vi "3654Drive2018.vi"(6 "turbo 2":bool, 7 "turbo 1":bool, 8 "Joystick2y":dbl, 9 "Joystick2x":dbl, 10 "joystick y":dbl, 11 "joystick x":dbl) -> ()   [LabVIEW 2017]
uses:
  <vilib>/Rock Robotics/WPI/ThirdParty/Phoenix-LabVIEW/Motor Controller/Controls/CTRE_Phoenix_MotorControl_ControlMode.ctl
  Robot Global Data.vi
  <vilib>/Rock Robotics/WPI/ThirdParty/Phoenix-LabVIEW/Motor Controller/Get/CTRE_Phoenix_MotorController_GetOutputCurrent_Enhanced.vi
  <vilib>/Rock Robotics/WPI/ThirdParty/Phoenix-LabVIEW/Motor Controller/Get/CTRE_Phoenix_MotorController_GetSelectedSensorData.vi
  <vilib>/Rock Robotics/WPI/ThirdParty/Phoenix-LabVIEW/Motor Controller/Get/CTRE_Phoenix_MotorController_GetClosedLoopData.vi
  <vilib>/Rock Robotics/WPI/ThirdParty/Phoenix-LabVIEW/Motor Controller/Get/CTRE_Phoenix_MotorController_GetVoltage.vi
panel:
  out "LeftCurrent":dbl
  out "RightCurrent":dbl
  out "RightClosed-loop Error":i32
  out "RightClosed-loop Target":i32
  out "LeftClosed-loop Error":i32
  out "LeftClosed-loop Target":i32
  out "RightSensorPosRotations":i32
  out "Motor output Plot 2":cluster{"Applied Throttle":dbl}(graph)
  out "RightTarget RPM":dbl
  out "RightSensorRPM Velocity RPM":i32
  out "RightApplied Output":dbl
  out "LeftSensorPosRotation":i32
  out "Motor output Plot":cluster{"Applied Throttle":dbl}(graph)
  out "LeftTarget RPM":dbl
  out "LeftSensorRPM Velocity RPM":i32
  out "LeftApplied Output":dbl
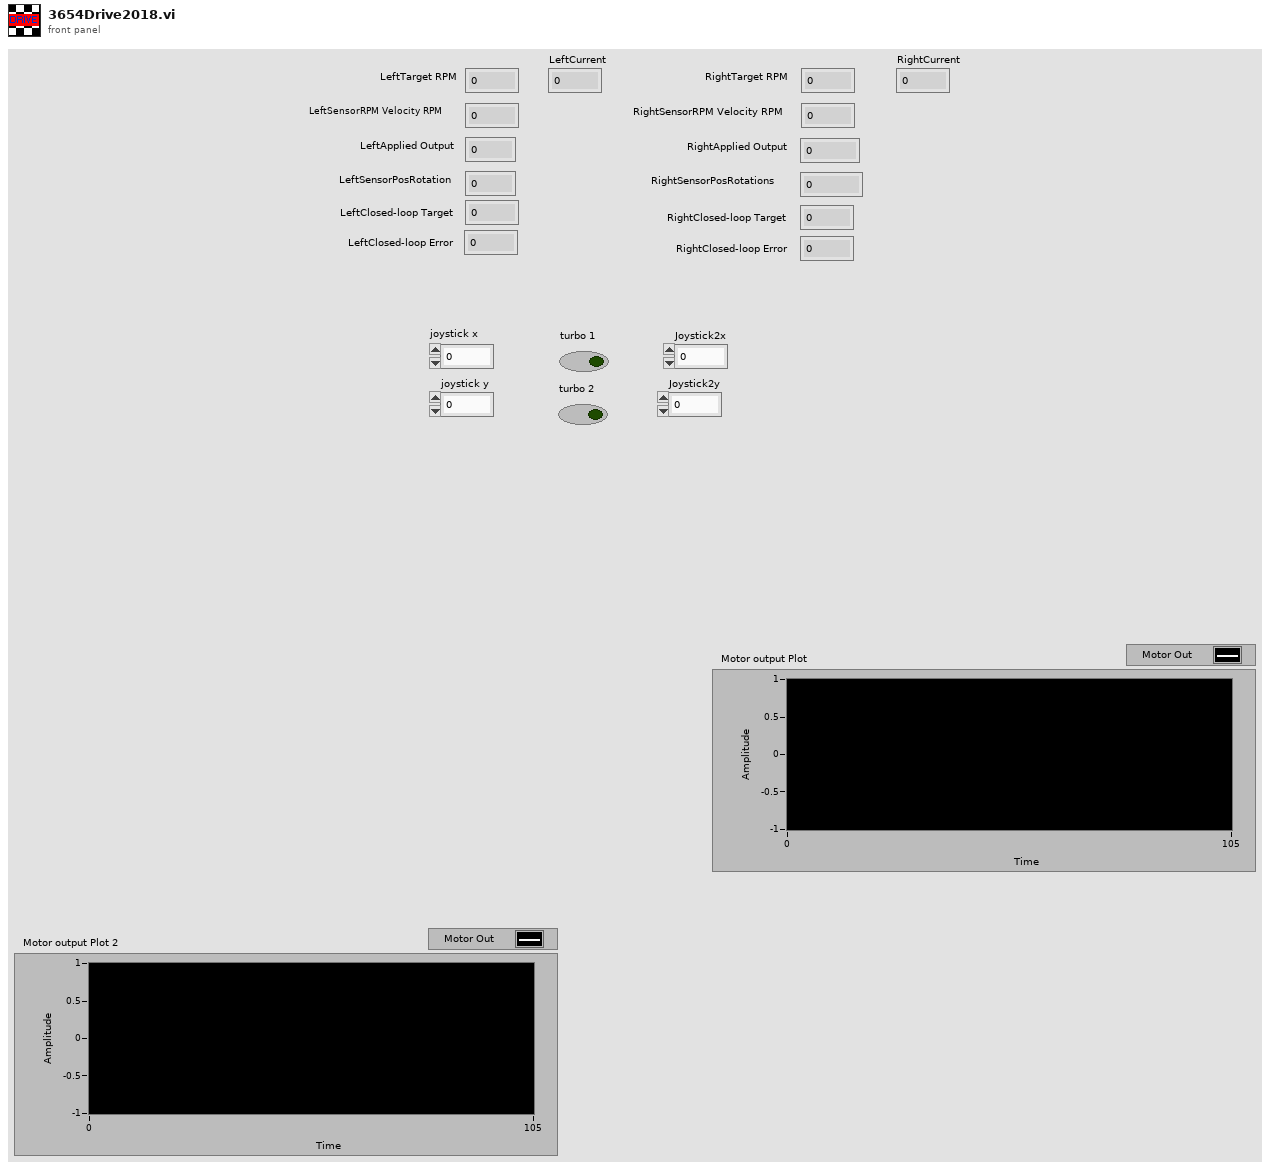
[diagram p1: front panel]
types:
  T1 = typedef "Encoder.ctl" = enum16{"NoEncoders", "ShaftEncoders", "MotorEncoders"}
  T2 = typedef "CTRE_Phoenix_MotorControl_ControlMode.ctl" = u16
  T3 = typedef "WPI_MotorControlDeviceRef.ctl" = cluster{"DeviceStatus":errorcluster, "Type":T4, "PWM":cluster{"PWM Channel":T5, "DeadBand":T6}, "CAN":cluster{"Device Number":u8, "SetOutput VI Ref":variant, "GetOutput VI Ref":variant, "Enable VI Ref":variant, "Disable VI Ref":variant, "Data":variant}, "Invert":bool, "DIO PWM":cluster{"PWM \"Enable\" Channel":T5, "DIOChannel":T7, "PWM Rate":dbl}}
  T4 = typedef "WPI_MotorControlType.ctl" = enum16{"PWM", "CAN", "DIO PWM"}
  T5 = typedef "FPGA_DIOPWMChannel.ctl" = enum8{"PWM 0", "PWM 1", "PWM 2", "PWM 3", "PWM 4", "PWM 5", "PWM 6", "PWM 7", "PWM 8", "PWM 9", "PWM MXP 0", "PWM MXP 1", "PWM MXP 2", "PWM MXP 3", "PWM MXP 4", "PWM MXP 5", "PWM MXP 6", "PWM MXP 7", "PWM MXP 8", "PWM MXP 9", "Invalid"}
  T6 = typedef "WPI_PWMDeadband.ctl" = cluster{"Name":string, "maxPositivePwm":i32, "minPositivePwm":i32, "centerPwm":i32, "maxNegativePwm":i32, "minNegativePwm":i32, "angularRange":u16}
  T7 = typedef "FPGA_DIOChannel.ctl" = enum8{"DIO 0", "DIO 1", "DIO 2", "DIO 3", "DIO 4", "DIO 5", "DIO 6", "DIO 7", "DIO 8", "DIO 9", "DIO MXP 0", "DIO MXP 1", "DIO MXP 2", "DIO MXP 3", "DIO MXP 4", "DIO MXP 5", "DIO MXP 6", "DIO MXP 7", "DIO MXP 8", "DIO MXP 9", "DIO MXP 10", "DIO MXP 11", "DIO MXP 12", "DIO MXP 13", "DIO MXP 14", "DIO MXP 15", "SPI Port CS1", "SPI Port CS2", "SPI Port CS3", "SPI Port MISO", "SPI Port MOSI", "Invalid"}
  T8 = typedef "DriveMode.ctl" = enum16{"1JoystickArcade", "2JoystickArcade", "Tank"}
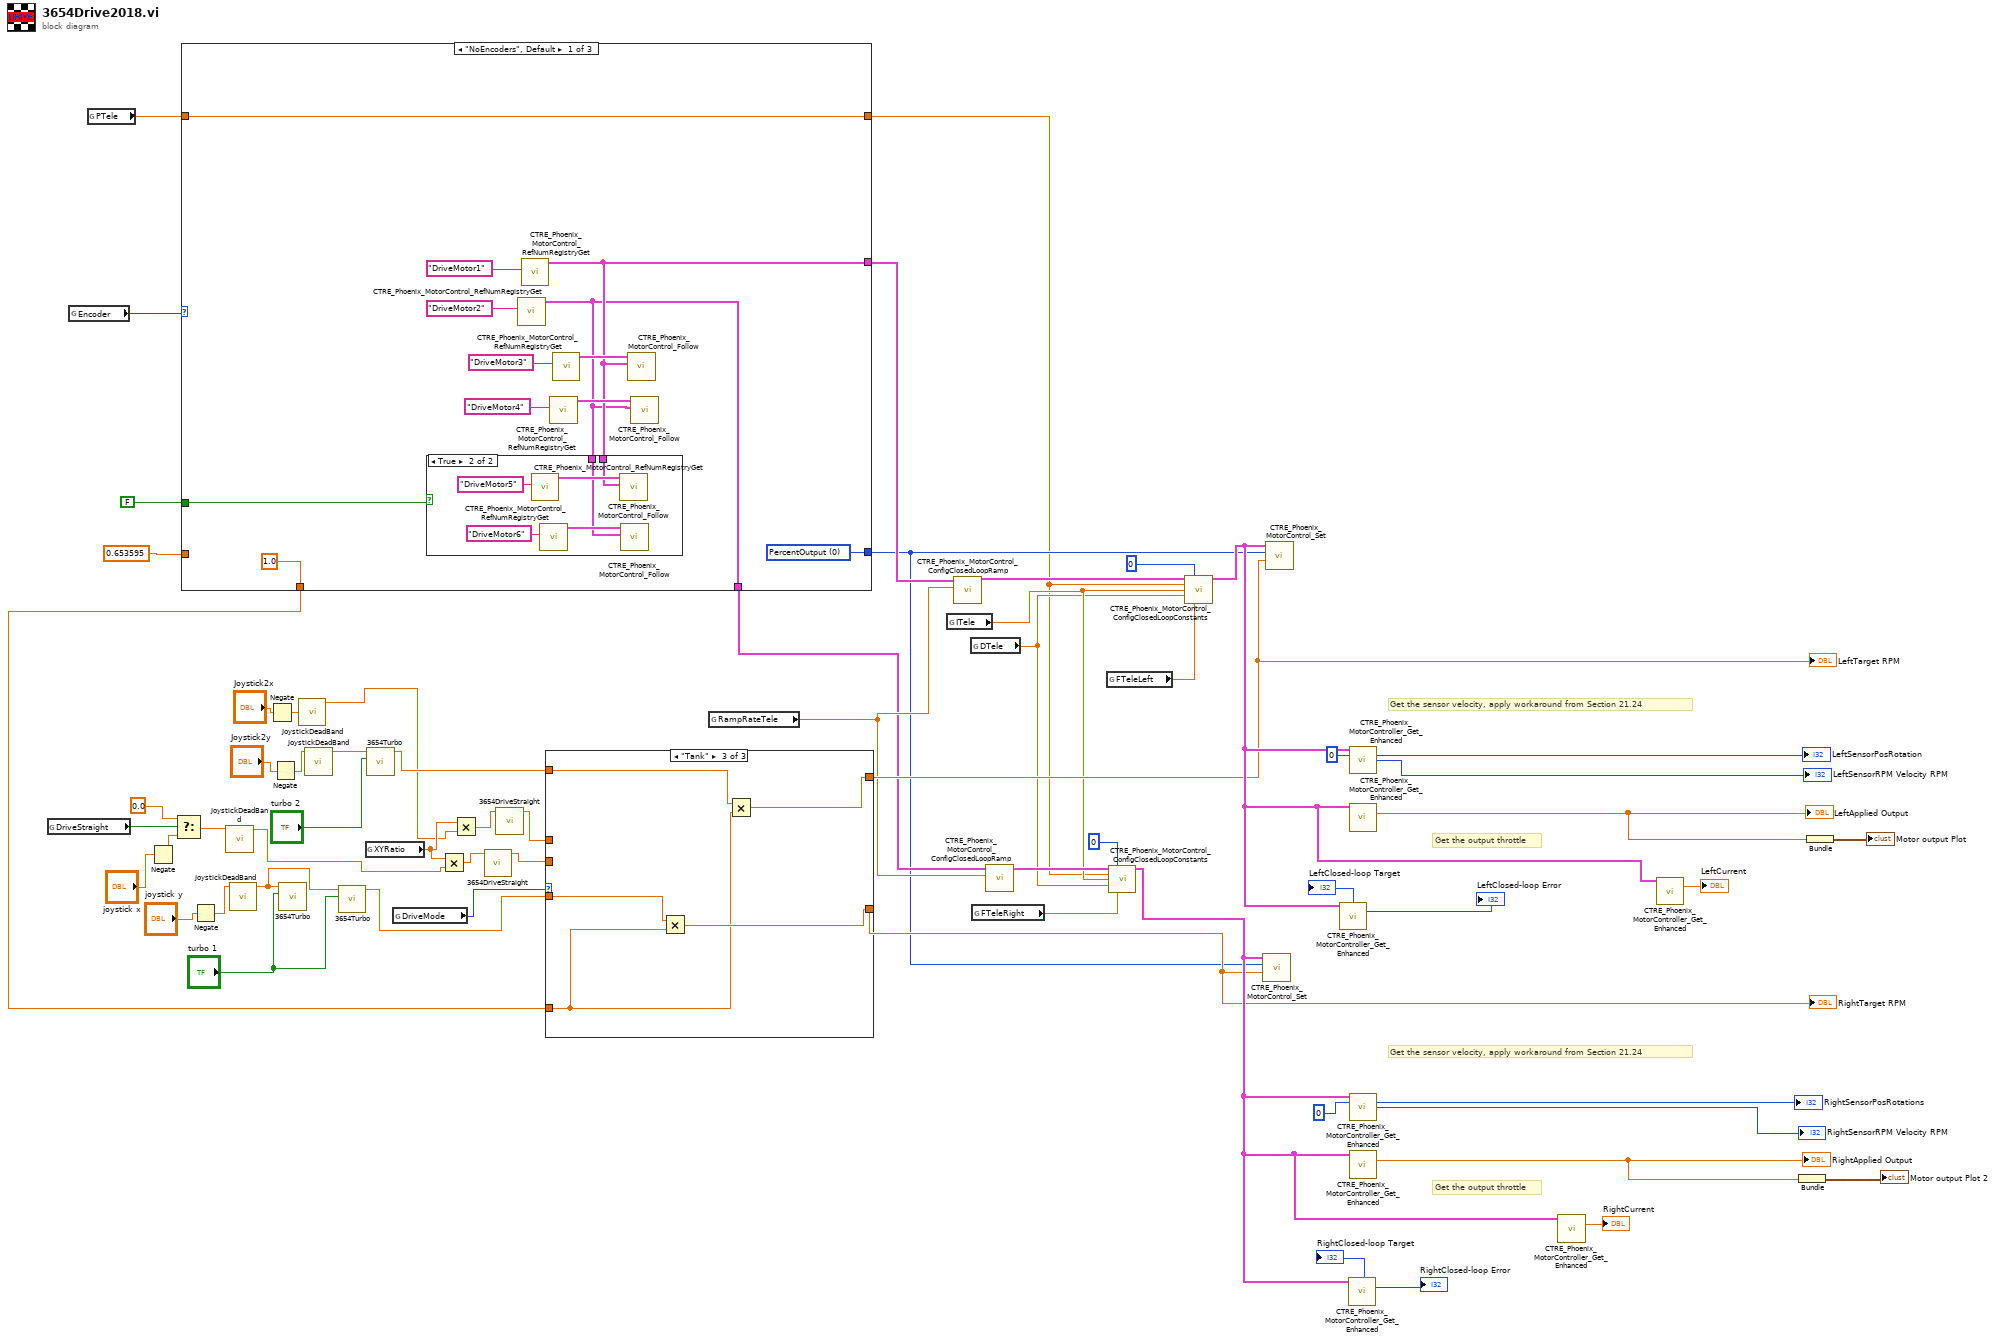
[diagram p0: block diagram]
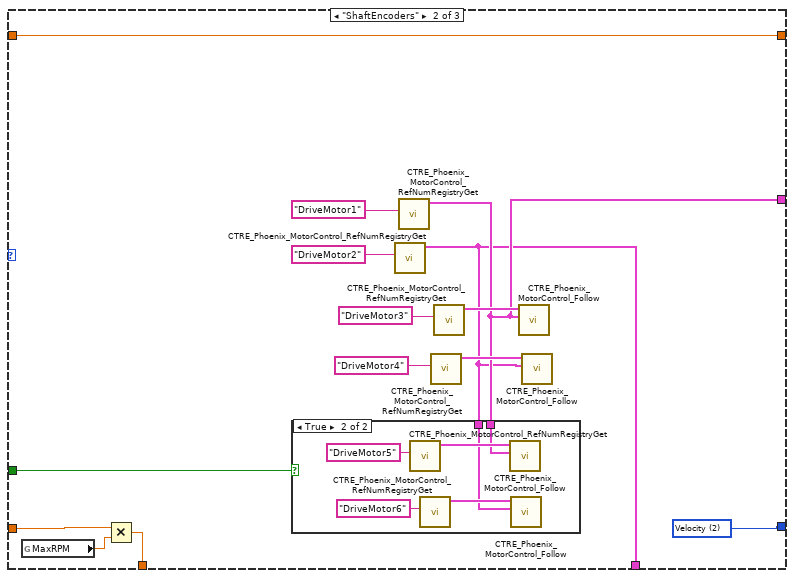
[diagram p3: hidden frame]
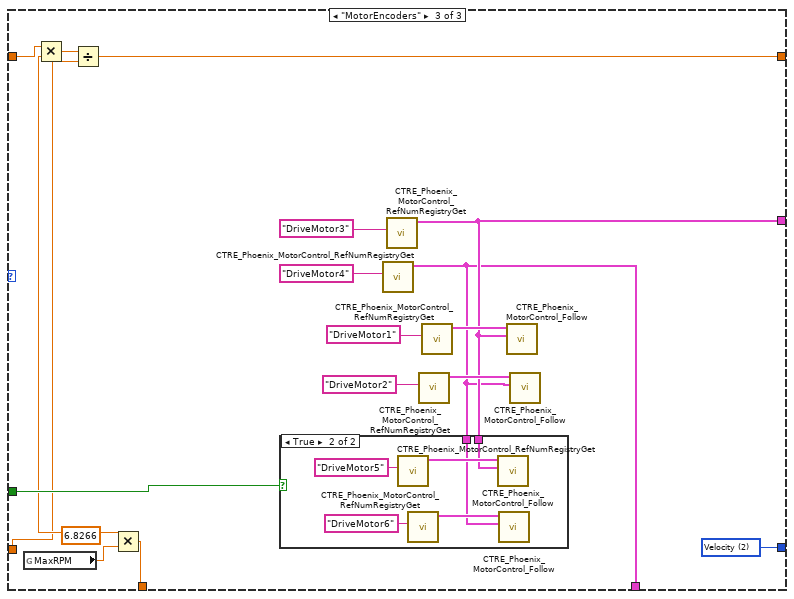
[diagram p5: hidden frame]
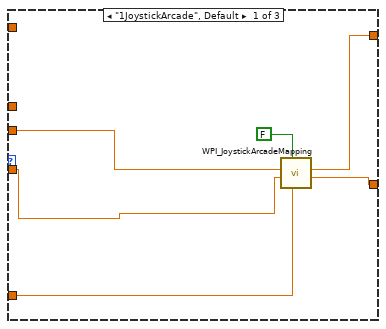
[diagram p7: hidden frame]
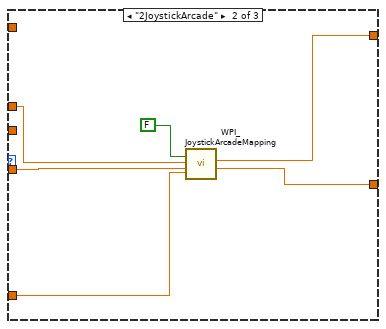
[diagram p8: hidden frame]
diagram:
  # "Get the output throttle"
  # "Get the sensor velocity, apply workaround from Section 21.24"
  # "Get the output throttle"
  # "Get the sensor velocity, apply workaround from Section 21.24"
  n1 = global read "Robot Global Data.vi" "DriveStraight"() -> (w41:bool)
  n2 = global read "Robot Global Data.vi" "Encoder"() -> (w10:T1)
  n3 = global read "Robot Global Data.vi" "PTele"() -> (w3:dbl)
  n4 = Negate(x="joystick x") -> (-x=w32:dbl)
  n5 = Select(t=0.0, s=w41, f=w32) -> (s? t:f=w40:dbl)
  n6 = case shown="\"NoEncoders\", Default" w10 {
    tunnel: [1.0 w94 w117] -> w8
    tunnel: [w74 w93 w116] -> w4
    tunnel: FALSE -> [w67 w86 w109]
    tunnel: [w66 w85 w108] -> w6
    tunnel: [w65 w84 w107] -> w5
    tunnel: w3 -> [w64 w83 w106]
    tunnel: [w64 w83 w102] -> w2
    tunnel: 0.653595 ("f") -> [_ w82 w103]
    frame "NoEncoders", Default {
      w74 = T2 0 items=["PercentOutput"=0, "Position"=1, "Velocity"=2, "Current"=3, "Follower"=5, "MotionProfile"=6, "MotionMagic"=7, "MotionMagicArc"=8, "MotionProfileArc"=10, "Disabled"=15] ("Control Mode")
      n7 = call <vilib>:"CTRE_Phoenix_MotorControl_RefNumRegistryGet.vi"("refnum name"="DriveMotor2") -> ("PhoenixMotorControlDevRef"=w65:T3)  [unwired: 9 in, 1 out]
      n8 = call <vilib>:"CTRE_Phoenix_MotorControl_RefNumRegistryGet.vi"("refnum name"="DriveMotor1") -> ("PhoenixMotorControlDevRef"=w66:T3)  [unwired: 9 in, 1 out]
      n9 = case shown="True" w67 {
        tunnel: w66 -> [_ w77]
        tunnel: w65 -> [_ w76]
        frame False {
        }
        frame True {
          n10 = call <vilib>:"CTRE_Phoenix_MotorControl_RefNumRegistryGet.vi"("refnum name"="DriveMotor5") -> ("PhoenixMotorControlDevRef"=w79:T3)  [unwired: 9 in, 1 out]
          n11 = call <vilib>:"CTRE_Phoenix_MotorControl_RefNumRegistryGet.vi"("refnum name"="DriveMotor6") -> ("PhoenixMotorControlDevRef"=w78:T3)  [unwired: 9 in, 1 out]
          n12 = call <vilib>:"CTRE_Phoenix_MotorControl_Follow.vi"("Master Controller to Follow"=w77, "PhoenixMotorControlDevRef"=w79) -> ()  [unwired: 8 in, 2 out]
          n13 = call <vilib>:"CTRE_Phoenix_MotorControl_Follow.vi"("Master Controller to Follow"=w76, "PhoenixMotorControlDevRef"=w78) -> ()  [unwired: 8 in, 2 out]
        }
      }
      n14 = call <vilib>:"CTRE_Phoenix_MotorControl_RefNumRegistryGet.vi"("refnum name"="DriveMotor4") -> ("PhoenixMotorControlDevRef"=w69:T3)  [unwired: 9 in, 1 out]
      n15 = call <vilib>:"CTRE_Phoenix_MotorControl_RefNumRegistryGet.vi"("refnum name"="DriveMotor3") -> ("PhoenixMotorControlDevRef"=w68:T3)  [unwired: 9 in, 1 out]
      n16 = call <vilib>:"CTRE_Phoenix_MotorControl_Follow.vi"("Master Controller to Follow"=w66, "PhoenixMotorControlDevRef"=w68) -> ()  [unwired: 8 in, 2 out]
      n17 = call <vilib>:"CTRE_Phoenix_MotorControl_Follow.vi"("Master Controller to Follow"=w65, "PhoenixMotorControlDevRef"=w69) -> ()  [unwired: 8 in, 2 out]
    }
    frame "ShaftEncoders" {
      w93 = T2 2 items=["PercentOutput"=0, "Position"=1, "Velocity"=2, "Current"=3, "Follower"=5, "MotionProfile"=6, "MotionMagic"=7, "MotionMagicArc"=8, "MotionProfileArc"=10, "Disabled"=15] ("Control Mode")
      n18 = global read "Robot Global Data.vi" "MaxRPM"() -> (w95:dbl)
      n19 = Multiply(x=w82, y=w95) -> (x*y=w94:dbl)
      n20 = call <vilib>:"CTRE_Phoenix_MotorControl_RefNumRegistryGet.vi"("refnum name"="DriveMotor2") -> ("PhoenixMotorControlDevRef"=w84:T3)  [unwired: 9 in, 1 out]
      n21 = call <vilib>:"CTRE_Phoenix_MotorControl_RefNumRegistryGet.vi"("refnum name"="DriveMotor1") -> ("PhoenixMotorControlDevRef"=w85:T3)  [unwired: 9 in, 1 out]
      n22 = case shown="True" w86 {
        tunnel: w85 -> [_ w97]
        tunnel: w84 -> [_ w96]
        frame False {
        }
        frame True {
          n23 = call <vilib>:"CTRE_Phoenix_MotorControl_RefNumRegistryGet.vi"("refnum name"="DriveMotor5") -> ("PhoenixMotorControlDevRef"=w99:T3)  [unwired: 9 in, 1 out]
          n24 = call <vilib>:"CTRE_Phoenix_MotorControl_RefNumRegistryGet.vi"("refnum name"="DriveMotor6") -> ("PhoenixMotorControlDevRef"=w98:T3)  [unwired: 9 in, 1 out]
          n25 = call <vilib>:"CTRE_Phoenix_MotorControl_Follow.vi"("Master Controller to Follow"=w97, "PhoenixMotorControlDevRef"=w99) -> ()  [unwired: 8 in, 2 out]
          n26 = call <vilib>:"CTRE_Phoenix_MotorControl_Follow.vi"("Master Controller to Follow"=w96, "PhoenixMotorControlDevRef"=w98) -> ()  [unwired: 8 in, 2 out]
        }
      }
      n27 = call <vilib>:"CTRE_Phoenix_MotorControl_RefNumRegistryGet.vi"("refnum name"="DriveMotor4") -> ("PhoenixMotorControlDevRef"=w88:T3)  [unwired: 9 in, 1 out]
      n28 = call <vilib>:"CTRE_Phoenix_MotorControl_RefNumRegistryGet.vi"("refnum name"="DriveMotor3") -> ("PhoenixMotorControlDevRef"=w87:T3)  [unwired: 9 in, 1 out]
      n29 = call <vilib>:"CTRE_Phoenix_MotorControl_Follow.vi"("Master Controller to Follow"=w85, "PhoenixMotorControlDevRef"=w87) -> ()  [unwired: 8 in, 2 out]
      n30 = call <vilib>:"CTRE_Phoenix_MotorControl_Follow.vi"("Master Controller to Follow"=w84, "PhoenixMotorControlDevRef"=w88) -> ()  [unwired: 8 in, 2 out]
    }
    frame "MotorEncoders" {
      w116 = T2 2 items=["PercentOutput"=0, "Position"=1, "Velocity"=2, "Current"=3, "Follower"=5, "MotionProfile"=6, "MotionMagic"=7, "MotionMagicArc"=8, "MotionProfileArc"=10, "Disabled"=15] ("Control Mode")
      w105 = 6.8266 ("Max Output")
      n31 = global read "Robot Global Data.vi" "MaxRPM"() -> (w118:dbl)
      n32 = Multiply(x=w106, y=w105) -> (x*y=w104:dbl)
      n33 = Divide(x=w104, y=w103) -> (x/y=w102:dbl)
      n34 = Multiply(x=w105, y=w118) -> (x*y=w117:dbl)
      n35 = call <vilib>:"CTRE_Phoenix_MotorControl_RefNumRegistryGet.vi"("refnum name"="DriveMotor4") -> ("PhoenixMotorControlDevRef"=w107:T3)  [unwired: 9 in, 1 out]
      n36 = call <vilib>:"CTRE_Phoenix_MotorControl_RefNumRegistryGet.vi"("refnum name"="DriveMotor3") -> ("PhoenixMotorControlDevRef"=w108:T3)  [unwired: 9 in, 1 out]
      n37 = case shown="True" w109 {
        tunnel: w108 -> [_ w120]
        tunnel: w107 -> [_ w119]
        frame False {
        }
        frame True {
          n38 = call <vilib>:"CTRE_Phoenix_MotorControl_RefNumRegistryGet.vi"("refnum name"="DriveMotor5") -> ("PhoenixMotorControlDevRef"=w122:T3)  [unwired: 9 in, 1 out]
          n39 = call <vilib>:"CTRE_Phoenix_MotorControl_RefNumRegistryGet.vi"("refnum name"="DriveMotor6") -> ("PhoenixMotorControlDevRef"=w121:T3)  [unwired: 9 in, 1 out]
          n40 = call <vilib>:"CTRE_Phoenix_MotorControl_Follow.vi"("Master Controller to Follow"=w120, "PhoenixMotorControlDevRef"=w122) -> ()  [unwired: 8 in, 2 out]
          n41 = call <vilib>:"CTRE_Phoenix_MotorControl_Follow.vi"("Master Controller to Follow"=w119, "PhoenixMotorControlDevRef"=w121) -> ()  [unwired: 8 in, 2 out]
        }
      }
      n42 = call <vilib>:"CTRE_Phoenix_MotorControl_RefNumRegistryGet.vi"("refnum name"="DriveMotor2") -> ("PhoenixMotorControlDevRef"=w111:T3)  [unwired: 9 in, 1 out]
      n43 = call <vilib>:"CTRE_Phoenix_MotorControl_RefNumRegistryGet.vi"("refnum name"="DriveMotor1") -> ("PhoenixMotorControlDevRef"=w110:T3)  [unwired: 9 in, 1 out]
      n44 = call <vilib>:"CTRE_Phoenix_MotorControl_Follow.vi"("Master Controller to Follow"=w108, "PhoenixMotorControlDevRef"=w110) -> ()  [unwired: 8 in, 2 out]
      n45 = call <vilib>:"CTRE_Phoenix_MotorControl_Follow.vi"("Master Controller to Follow"=w107, "PhoenixMotorControlDevRef"=w111) -> ()  [unwired: 8 in, 2 out]
    }
  }
  n46 = Negate(x="joystick y") -> (-x=w35:dbl)
  n47 = call "JoystickDeadBand.vi"("JoystickInput"=w40) -> ("JoystickAfterDeadband"=w23:dbl)  [unwired: 10 in]
  n48 = call "JoystickDeadBand.vi"("JoystickInput"=w35) -> ("JoystickAfterDeadband"=w18:dbl)  [unwired: 10 in]
  n49 = Negate(x="Joystick2x") -> (-x=w28:dbl)
  n50 = Negate(x="Joystick2y") -> (-x=w30:dbl)
  n51 = call "3654Turbo.vi"("ButtonPressed?"="turbo 1", "Input"=w18) -> ()  [unwired: 9 in, 1 out]
  n52 = call "JoystickDeadBand.vi"("JoystickInput"=w28) -> ("JoystickAfterDeadband"=w24:dbl)  [unwired: 10 in]
  n53 = call "JoystickDeadBand.vi"("JoystickInput"=w30) -> ("JoystickAfterDeadband"=w53:dbl)  [unwired: 10 in]
  n54 = call "3654Turbo.vi"("ButtonPressed?"="turbo 1", "Input"=w18) -> ("Output"=w20:dbl)  [unwired: 9 in]
  n55 = global read "Robot Global Data.vi" "XYRatio"() -> (w27:dbl)
  n56 = call "3654Turbo.vi"("ButtonPressed?"="turbo 2", "Input"=w53) -> ("Output"=w47:dbl)  [unwired: 9 in]
  n57 = global read "Robot Global Data.vi" "DriveMode"() -> (w9:T8)
  n58 = Multiply(x=w27, y=w23) -> (x*y=w26:dbl)
  n59 = Multiply(x=w27, y=w24) -> (x*y=w22:dbl)
  n60 = call "3654DriveStraight.vi"("X-AxisIn"=w26) -> ("X-AxisOut"=w25:dbl)  [unwired: 10 in]
  n61 = call "3654DriveStraight.vi"("X-AxisIn"=w22) -> ("X-AxisOut"=w21:dbl)  [unwired: 10 in]
  n62 = case shown="\"Tank\"" w9 {
    tunnel: [w129 w132 w140] -> w16
    tunnel: [w130 w131 w137] -> w36
    tunnel: w20 -> [w127 w133 w141]
    tunnel: w25 -> [w128 _ _]
    tunnel: w47 -> [_ _ w138]
    tunnel: w21 -> [_ w135 _]
    tunnel: w8 -> [w125 w134 w139]
    frame "1JoystickArcade", Default {
      n63 = call <vilib>:"WPI_JoystickArcadeMapping.vi"("Max Output"=w125, "Square Inputs"=FALSE, "Y axis value"=w127, "X axis value"=w128) -> ("Right Motor Value"=w129:dbl, "Left Motor Value"=w130:dbl)  [unwired: 6 in]
    }
    frame "2JoystickArcade" {
      n64 = call <vilib>:"WPI_JoystickArcadeMapping.vi"("Max Output"=w134, "Square Inputs"=FALSE, "Y axis value"=w133, "X axis value"=w135) -> ("Right Motor Value"=w132:dbl, "Left Motor Value"=w131:dbl)  [unwired: 6 in]
    }
    frame "Tank" {
      n65 = Multiply(x=w141, y=w139) -> (x*y=w140:dbl)
      n66 = Multiply(x=w138, y=w139) -> (x*y=w137:dbl)
    }
  }
  "LeftTarget RPM" <- w36
  "RightTarget RPM" <- w16
  n67 = global read "Robot Global Data.vi" "RampRateTele"() -> (w11:dbl)
  n68 = global read "Robot Global Data.vi" "ITele"() -> (w13:dbl)
  n69 = call <vilib>:"CTRE_Phoenix_MotorControl_ConfigClosedLoopRamp.vi"("secondsFromNeutralToFull"=w11, "PhoenixMotorControlDevRef"=w6) -> ("PhoenixMotorControlDevRef"=w45:T3)  [unwired: 8 in, 1 out]
  n70 = global read "Robot Global Data.vi" "DTele"() -> (w12:dbl)
  n71 = global read "Robot Global Data.vi" "FTeleRight"() -> (w15:dbl)
  n72 = call <vilib>:"CTRE_Phoenix_MotorControl_ConfigClosedLoopRamp.vi"("secondsFromNeutralToFull"=w11, "PhoenixMotorControlDevRef"=w5) -> ("PhoenixMotorControlDevRef"=w43:T3)  [unwired: 8 in, 1 out]
  n73 = global read "Robot Global Data.vi" "FTeleLeft"() -> (w14:dbl)
  n74 = call <vilib>:"CTRE_Phoenix_MotorControl_ConfigClosedLoopConstants.vi"("PhoenixMotorControlDevRef"=w43, "slotIdx"=0, "P"=w2, "I"=w13, "D"=w12, "F"=w15) -> ("PhoenixMotorControlDevRef"=w17:T3)  [unwired: 8 in, 1 out]
  n75 = call <vilib>:"CTRE_Phoenix_MotorControl_ConfigClosedLoopConstants.vi"("PhoenixMotorControlDevRef"=w45, "slotIdx"=0, "P"=w2, "I"=w13, "D"=w12, "F"=w14) -> ("PhoenixMotorControlDevRef"=w39:T3)  [unwired: 8 in, 1 out]
  n76 = call <vilib>:"CTRE_Phoenix_MotorControl_Set.vi"("Output"=w16, "Control Mode"=w4, "PhoenixMotorControlDevRef"=w17) -> ()  [unwired: 7 in, 2 out]
  n77 = call <vilib>:"CTRE_Phoenix_MotorControl_Set.vi"("Output"=w36, "Control Mode"=w4, "PhoenixMotorControlDevRef"=w39) -> ()  [unwired: 7 in, 2 out]
  n78 = call-poly <vilib>:"CTRE_Phoenix_MotorController_Get_Enhanced.vi"("PhoenixMotorControlDevRef"=w39) -> ("Closed-loop Target"=→"LeftClosed-loop Target":i32, "Closed-loop Error"=→"LeftClosed-loop Error":i32)  [unwired: 9 in, 4 out]
  n79 = call-poly <vilib>:"CTRE_Phoenix_MotorController_Get_Enhanced.vi"("PhoenixMotorControlDevRef"=w17) -> ("Closed-loop Target"=→"RightClosed-loop Target":i32, "Closed-loop Error"=→"RightClosed-loop Error":i32)  [unwired: 9 in, 4 out]
  n80 = call-poly <vilib>:"CTRE_Phoenix_MotorController_Get_Enhanced.vi"("PhoenixMotorControlDevRef"=w39, "pidLoopIdx"=u32 0) -> ("Position (Raw Sensor Units)"=→"LeftSensorPosRotation":i32, "Velocity (Raw Sensor Units per 100 ms)"=→"LeftSensorRPM Velocity RPM":i32)  [unwired: 10 in, 2 out]
  n81 = call-poly <vilib>:"CTRE_Phoenix_MotorController_Get_Enhanced.vi"("PhoenixMotorControlDevRef"=w39) -> ("Percent Output"=w60:dbl)  [unwired: 10 in, 4 out]
  "LeftApplied Output" <- w60
  n82 = call-poly <vilib>:"CTRE_Phoenix_MotorController_Get_Enhanced.vi"("PhoenixMotorControlDevRef"=w17, "pidLoopIdx"=u32 0) -> ("Position (Raw Sensor Units)"=→"RightSensorPosRotations":i32, "Velocity (Raw Sensor Units per 100 ms)"=→"RightSensorRPM Velocity RPM":i32)  [unwired: 10 in, 2 out]
  n83 = call-poly <vilib>:"CTRE_Phoenix_MotorController_Get_Enhanced.vi"("PhoenixMotorControlDevRef"=w17) -> ("Percent Output"=w55:dbl)  [unwired: 10 in, 4 out]
  "RightApplied Output" <- w55
  n84 = call-poly <vilib>:"CTRE_Phoenix_MotorController_Get_Enhanced.vi"("PhoenixMotorControlDevRef"=w17) -> ("Output Current"=→"RightCurrent":dbl)  [unwired: 12 in, 2 out]
  n85 = call-poly <vilib>:"CTRE_Phoenix_MotorController_Get_Enhanced.vi"("PhoenixMotorControlDevRef"=w39) -> ("Output Current"=→"LeftCurrent":dbl)  [unwired: 12 in, 2 out]
  n86 = Bundle("Percent Output"=w55) -> (→"Motor output Plot 2":cluster{"Percent Output":dbl})  [unwired: 1 in]
  n87 = Bundle("Percent Output"=w60) -> (→"Motor output Plot":cluster{"Percent Output":dbl})  [unwired: 1 in]
